vi "SetBeads.vi"(0 "IntGraph Refnum":refnum<vi>, 1 "Autofind":bool, 2 "Add bead":bool, 3 "load beadlist":bool, 5 "save beadlist":bool, 8 "Reset all":bool, 9 "Remove bead #":bool, 11 "bead number":i32) -> (10 "Bead Array":i32[][](array[numeric]))   [LabVIEW 2011]
uses:
  <vilib>/Utility/file.llb/Read From Spreadsheet File (DBL).vi
  <vilib>/Utility/file.llb/Write To Spreadsheet File (DBL).vi
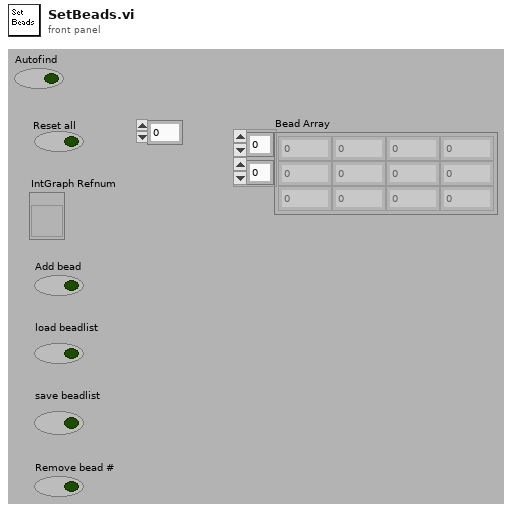
[diagram p1: front panel]
types:
  T1 = typedef "IMAQ Image.ctl" = refnum<image>
  T2 = cluster{"front panel settings":cluster{"files":cluster{"LUT path":path, "Trace path":path, " folders #":i32, "base path":path, "use trace":bool, "use base":bool, "LUT tmp":i32, "Trace tmp":i32, "active path":path}, "Tracking":cluster{"RminZ (pix)":i32, "Rmax (pix)":i32, "angular pixel \ncoverage factor":dbl, "radial pixel \ncoverage factor":dbl}, "Frames":cluster{"Start frame":i32, "number of frames":u32, "display frame ":i32, "track every nd frame ":i32, "Track all frames":bool, "active frame":i32}, "Calibs":cluster{"Zlut number of steps":i32, "pix/um":dbl, "Z correction factor":dbl, "Zlut step size (um)":dbl, "ROI(pix)":i32}, "Beads":cluster{"number of ref beads":i32, "overlay":bool}, "Misc":cluster{"save images to new location":bool, "destination":path}}, "data":cluster{"Image":T1, "image size":i32[], "Bead Array":i32[][], "overlay image":T1, "# beads":i32, "Job list":string[][], "job running":bool, "job #":i32, "folders to go":i32}}
  T3 = typedef "LVPointDoubleTypeDef.ctl" = cluster{"Cursor X":dbl, "Cursor Y":dbl}
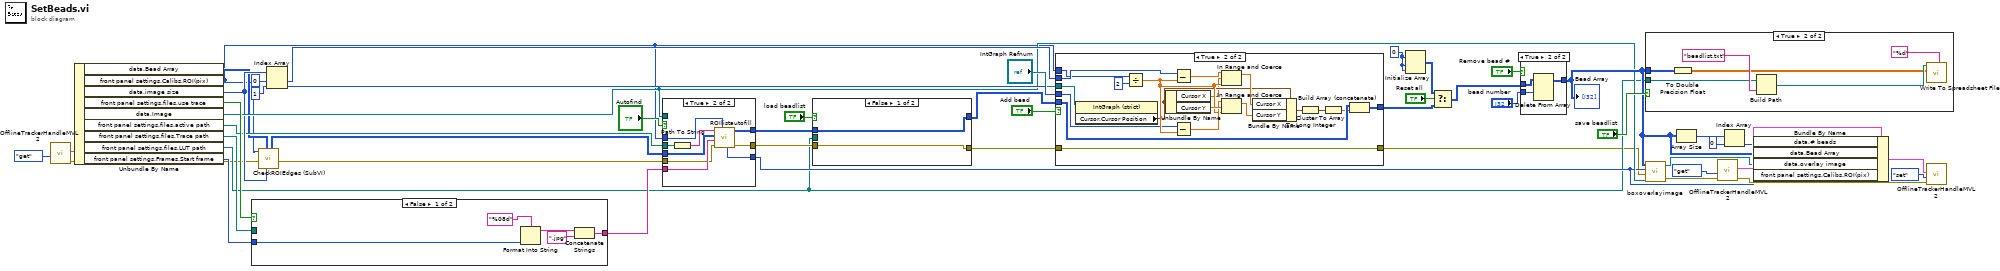
[diagram p0: block diagram]
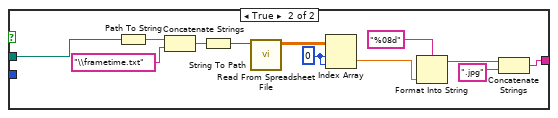
[diagram p2: hidden frame]
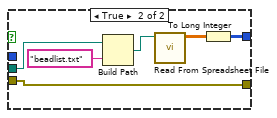
[diagram p6: hidden frame]
diagram:
  w38 = 0 ("element")
  n1 = call "OfflineTrackerHandleMVL2.vi"("action"=enum16{"get", "set"}."get") -> ("error out"=w5:errorcluster, "out"=w26:T2)  [unwired: 5 in]
  n2 = Unbundle By Name(w26) -> ("data.Bead Array"=w7:i32[][], "front panel settings.Calibs.ROI(pix)"=w1:i32, "data.image size"=w11:i32[], "front panel settings.files.use trace"=w14:bool, "data.Image"=w12:T1, "front panel settings.files.active path"=w10:path, "front panel settings.files.Trace path"=w25:path, "front panel settings.files.LUT path"=w8:path, "front panel settings.Frames.Start frame"=w13:i32)
  n3 = case shown="False" w14 {
    tunnel: w25 -> [_ w61]
    tunnel: [w50 w56] -> w23
    tunnel: w13 -> [w49 _]
    frame False {
      n4 = Format Into String(format string="%08d", w49) -> (resulting string=w52:string)  [unwired: 2 in, 1 out]
      n5 = Concatenate Strings(w52, ".jpg" ("string")) -> (w50:string)
    }
    frame True {
      w54 = 0 ("index")
      n6 = Path To String(path=w61) -> (string=w65:string)
      n7 = Concatenate Strings(w65, "\\frametime.txt" ("string")) -> (w63:string)
      n8 = String To Path(string=w63) -> (path=w64:path)
      n9 = call-poly <vilib>:"Read From Spreadsheet File.vi"("file path (dialog if empty)"=w64) -> ("all rows"=w55:dbl[][])  [unwired: 3 in, 7 out]
      n10 = Index Array(array=w55, index (row)=w54, index (col)=w54) -> (element=w60:dbl)
      n11 = Format Into String(format string="%08d", w60) -> (resulting string=w58:string)  [unwired: 2 in, 1 out]
      n12 = Concatenate Strings(w58, ".jpg" ("string")) -> (w56:string)
    }
  }
  n13 = call "CheckROIEdges (SubVI).vi"("image size"=w11, "Bead Array"=w7, "error out 2"=w5, "front panel settings.Calibs.ROI(pix)"=w1) -> ("error out"=w4:errorcluster, "Bead Array adapted"=w6:i32[][])  [unwired: 6 in]
  n14 = Index Array(array=w11, index #1=0 ("index"), index #2=1 ("index")) -> (element #1=w43:i32, element #2=w42:i32)
  n15 = case shown="True" "Autofind" {
    tunnel: [w68 w74] -> w30
    tunnel: w6 -> [w68 w71]
    tunnel: w12 -> [_ _]
    tunnel: w10 -> [_ w77]
    tunnel: w1 -> [w66 w75]
    tunnel: w23 -> [_ w73]
    tunnel: [w67 w72] -> w29
    tunnel: w4 -> [w67 w70]
    tunnel: [w66 w69] -> w9
    frame False {
    }
    frame True {
      n16 = Path To String(path=w77) -> (string=w76:string)
      n17 = call "ROIlistautofill.vi"("ROI in (pix)"=w75, "error out"=w70, "ImageName"=w73, "bead array in"=w71, "ImagePath"=w76) -> ("error out 2"=w72:errorcluster, "ROI center list"=w74:i32[][], "ROI out"=w69:i32)  [unwired: 4 out]
    }
  }
  n18 = case shown="False" "load beadlist" {
    tunnel: w30 -> [w79 _]
    tunnel: [w79 w84] -> w44
    tunnel: w29 -> [w78 w81]
    tunnel: [w78 w81] -> w28
    tunnel: w8 -> [_ w80]
    frame False {
    }
    frame True {
      n19 = Build Path(base path=w80, name or relative path="beadlist.txt") -> (appended path=w82:path)
      n20 = call-poly <vilib>:"Read From Spreadsheet File.vi"("file path (dialog if empty)"=w82) -> ("all rows"=w85:dbl[][])  [unwired: 3 in, 7 out]
      n21 = To Long Integer(number=w85) -> (32bit integer=w84:i32[][])
    }
  }
  n22 = case shown="True" "Add bead" {
    tunnel: [w87 w105] -> w39
    tunnel: w1 -> [_ w95]
    tunnel: w44 -> [w87 w98]
    tunnel: w42 -> [_ w97]
    tunnel: w43 -> [_ w96]
    tunnel: "IntGraph Refnum" -> [_ w89]
    tunnel: w28 -> [w86 w88]
    tunnel: [w86 w88] -> w3
    frame False {
    }
    frame True {
      n23 = property on="Property Node" class="IntGraph (strict)"(reference=w89) -> ("Cursor.Cursor Position"=w94:T3)  [unwired: 1 in, 2 out]
      n24 = Divide(x=w95, y=2) -> (x/y=w99:dbl)
      n25 = Unbundle By Name(w94) -> ("Cursor X"=w92:dbl, "Cursor Y"=w104:dbl)
      n26 = Subtract(x=w96, y=w99) -> (x-y=w101:dbl)
      n27 = Subtract(x=w97, y=w99) -> (x-y=w100:dbl)
      n28 = In Range and Coerce(upper limit=w101, x=w92, lower limit=w99) -> (coerced(x)=w103:dbl)  [unwired: 1 out]
      n29 = In Range and Coerce(upper limit=w100, x=w104, lower limit=w99) -> (coerced(x)=w102:dbl)  [unwired: 1 out]
      n30 = Bundle By Name(cluster=w94, "Cursor X"=w103, "Cursor Y"=w102) -> (w91:T3)
      n31 = To Long Integer(number=w91) -> (32bit integer=w93:cluster{"Cursor X":i32, "Cursor Y":i32})
      n32 = Cluster To Array(cluster=w93) -> (array=w90:i32[])
      n33 = Build Array (concatenate)(w98, w90) -> (w105:i32[][])
    }
  }
  n34 = Initialize Array(w38, w38, w38) -> (w36:i32[][])
  n35 = Select(t=w36, s="Reset all", f=w39) -> (s? t:f=w35:i32[][])
  n36 = case shown="True" "Remove bead #" {
    tunnel: [w107 w110] -> w18
    tunnel: w35 -> [w107 w109]
    tunnel: "bead number" -> [_ w108]
    frame False {
    }
    frame True {
      n37 = Delete From Array(array=w109, index (row)=w108) -> (array with subset deleted=w110:i32[][])  [unwired: 2 in, 1 out]
    }
  }
  "Bead Array" <- w18
  n38 = case shown="True" "save beadlist" {
    tunnel: w18 -> [_ w113]
    tunnel: w8 -> [_ w111]
    frame False {
    }
    frame True {
      n39 = To Double Precision Float(number=w113) -> (double precision float=w114:dbl[][])
      n40 = Build Path(base path=w111, name or relative path="beadlist.txt") -> (appended path=w115:path)
      n41 = call-poly <vilib>:"Write To Spreadsheet File.vi"("format (%.3f)"="%d", "2D data"=w114, "file path (dialog if empty)"=w115) -> ()  [unwired: 3 in, 3 out]
    }
  }
  n42 = call "boxoverlayimage.vi"("Image"=w12, "error in (no error)"=w3, "ROI"=w9, "Array"=w18) -> ("error out"=w2:errorcluster, "Image Out"=w17:T1)  [unwired: 1 out]
  n43 = Array Size(array=w18) -> (size(s)=w46:i32[])
  n44 = call "OfflineTrackerHandleMVL2.vi"("error in"=w2, "action"=enum16{"get", "set"}."get") -> ("error out"=w15:errorcluster, "out"=w20:T2)  [unwired: 4 in]
  n45 = Index Array(array=w46, index=0) -> (element=w19:i32)
  n46 = Bundle By Name(cluster=w20, "data.# beads"=w19, "data.Bead Array"=w18, "data.overlay image"=w17, "front panel settings.Calibs.ROI(pix)"=w9) -> (w16:T2)
  n47 = call "OfflineTrackerHandleMVL2.vi"("error in"=w15, "action"=enum16{"get", "set"}."set", "in"=w16) -> ()  [unwired: 3 in, 2 out]
